vi "get SetupComment.vi"(8 "error in (no error)":errorcluster caption="Fehler (Eingang, kein Fehler)", 11 "Setup (Eingang)":refnum<class "Setup.lvclass">) -> (0 "error out":errorcluster caption="Fehler (Ausgang)", 2 "Comment":string, 3 "Setup (Ausgang)":refnum<class "Setup.lvclass">)   [LabVIEW 2013, in "DatenKlassen.lvlib" / "Setup.lvclass"]
uses:
  Setup.lvclass
  Setup.lvclass/Setup.ctl
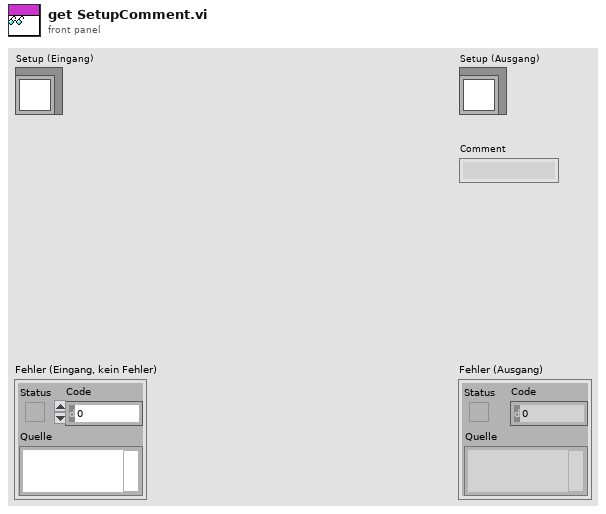
[diagram p1: front panel]
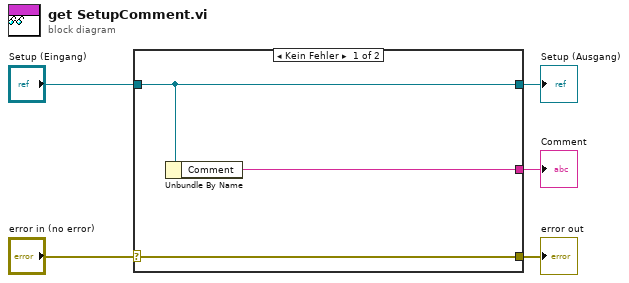
[diagram p0: block diagram]
diagram:
  n1 = case shown="Kein Fehler" "error in (no error)" {
    selector: "error in (no error)" -> [w8 w9]
    tunnel: [w8 w9] -> w4
    tunnel: [w7 w10] -> w2
    tunnel: "Setup (Eingang)" -> [w7 w10]
    tunnel: [w6 _] -> w1
    frame No Error {
      n2 = Unbundle By Name(w7) -> ("Comment"=w6:string)
    }
    frame Error {
    }
  }
  "error out" <- w4
  "Setup (Ausgang)" <- w2
  "Comment" <- w1
